vi "ixonScan.vi"(8 "stageReturnPosition":string, 9 "goBackAfterScan":bool=TRUE, 10 "scanStep":dbl, 11 "scanLength":dbl=25.0) -> (2 "Right Graph":i32[][](graph) caption="Object Image", 3 "imageCube":i32[][][](array[numeric]))   [LabVIEW 2016]
uses:
  <userlib>/atmcd64d.llb/Error Code Enum typedef.ctl
  <vilib>/Instr/_visa.llb/VISA Configure Serial Port (Instr).vi
  variables/imageSettings.vi
  variables/configDB.vi
panel:
  in  "Scan Abort":bool
  out "relative seconds 2":dbl format="%_19f"
  out "relative seconds":dbl format="%_19f"
  out "Constructing data":u8(slide) scale=0.0..256.0
  out "x-y":dbl
  out "Total \nScan Frame":dbl
  out "Current \nScan Frame":dbl
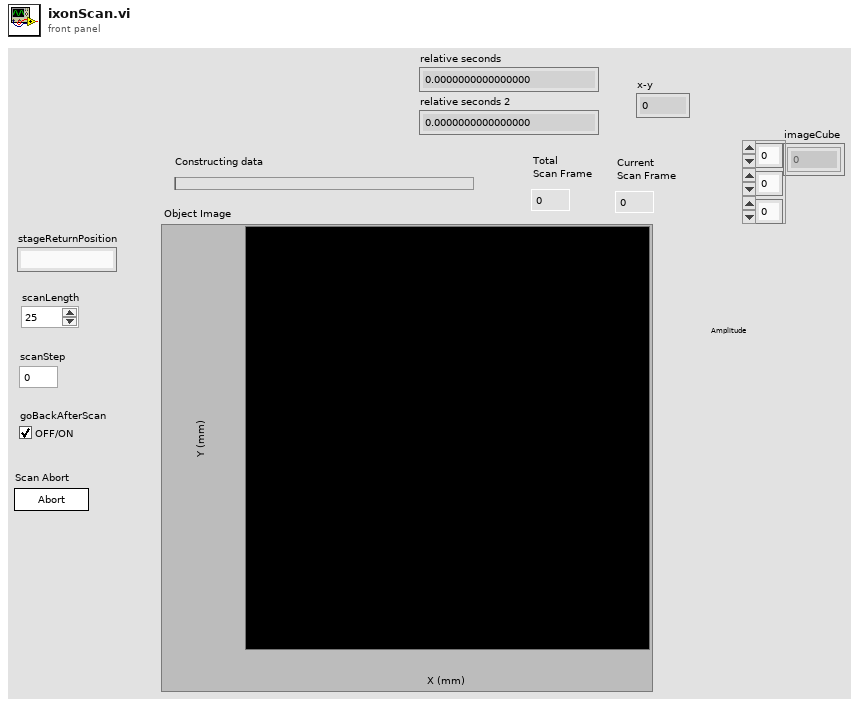
[diagram p1: front panel]
types:
  T1 = typedef "Error Code Enum typedef.ctl" = enum32{"N/A (0)", "DRV_ERROR_CODES", "DRV_SUCCESS", "DRV_VXDNOTINSTALLED", "DRV_ERROR_SCAN", "DRV_ERROR_CHECK_SUM", "DRV_ERROR_FILELOAD", "DRV_UNKNOWN_FUNC", "DRV_ERROR_VXD_INIT", "DRV_ERROR_ADDRESS", "DRV_ERROR_PAGELOCK", "DRV_ERROR_PAGEUNLOCK", "DRV_ERROR_BOARDTEST", "DRV_ERROR_ACK", "DRV_ERROR_UP_FIFO", "DRV_ERROR_PATTERN", "N/A (16)", "DRV_ACQUISITION_ERRORS", "DRV_ACQ_BUFFER", "DRV_ACQ_DOWNFIFO_FULL", "DRV_PROC_UNKONWN_INSTRUCTION", "DRV_ILLEGAL_OP_CODE", "DRV_KINETIC_TIME_NOT_MET", "DRV_ACCUM_TIME_NOT_MET", "DRV_NO_NEW_DATA", "N/A (25)", "DRV_SPOOLERROR", "N/A (27)", "N/A (28)", "N/A (29)", "N/A (30)", "N/A (31)", "N/A (32)", "DRV_TEMPERATURE_CODES", "DRV_TEMPERATURE_OFF", "DRV_TEMPERATURE_NOT_STABILIZED", "DRV_TEMPERATURE_STABILIZED", "DRV_TEMPERATURE_NOT_REACHED", "DRV_TEMPERATURE_OUT_RANGE", "DRV_TEMPERATURE_NOT_SUPPORTED", "DRV_TEMPERATURE_DRIFT", "N/A (41)", "N/A (42)", "N/A (43)", "N/A (44)", "N/A (45)", "N/A (46)", "N/A (47)", "N/A (48)", "DRV_GENERAL_ERRORS", "DRV_INVALID_AUX", "DRV_COF_NOTLOADED", "DRV_FPGAPROG", "DRV_FLEXERROR", "DRV_GPIBERROR", "N/A (55)", "N/A (56)", "N/A (57)", "N/A (58)", "N/A (59)", "N/A (60)", "N/A (61)", "N/A (62)", "N/A (63)", "DRV_DATATYPE", "DRV_DRIVER_ERRORS", "DRV_P1INVALID", "DRV_P2INVALID", "DRV_P3INVALID", "DRV_P4INVALID", "DRV_INIERROR", "DRV_COFERROR", "DRV_ACQUIRING", "DRV_IDLE", "DRV_TEMPCYCLE", "DRV_NOT_INITIALIZED", "DRV_P5INVALID", "DRV_P6INVALID", "DRV_INVALID_MODE", "DRV_INVALID_FILTER", "DRV_I2CERRORS", "DRV_I2CDEVNOTFOUND", "DRV_I2CTIMEOUT", "DRV_P7INVALID", "N/A (84)", "N/A (85)", "N/A (86)", "N/A (87)", "N/A (88)", "N/A (89)", "DRV_IOCERROR", "DRV_VRMVERSIONERROR"}
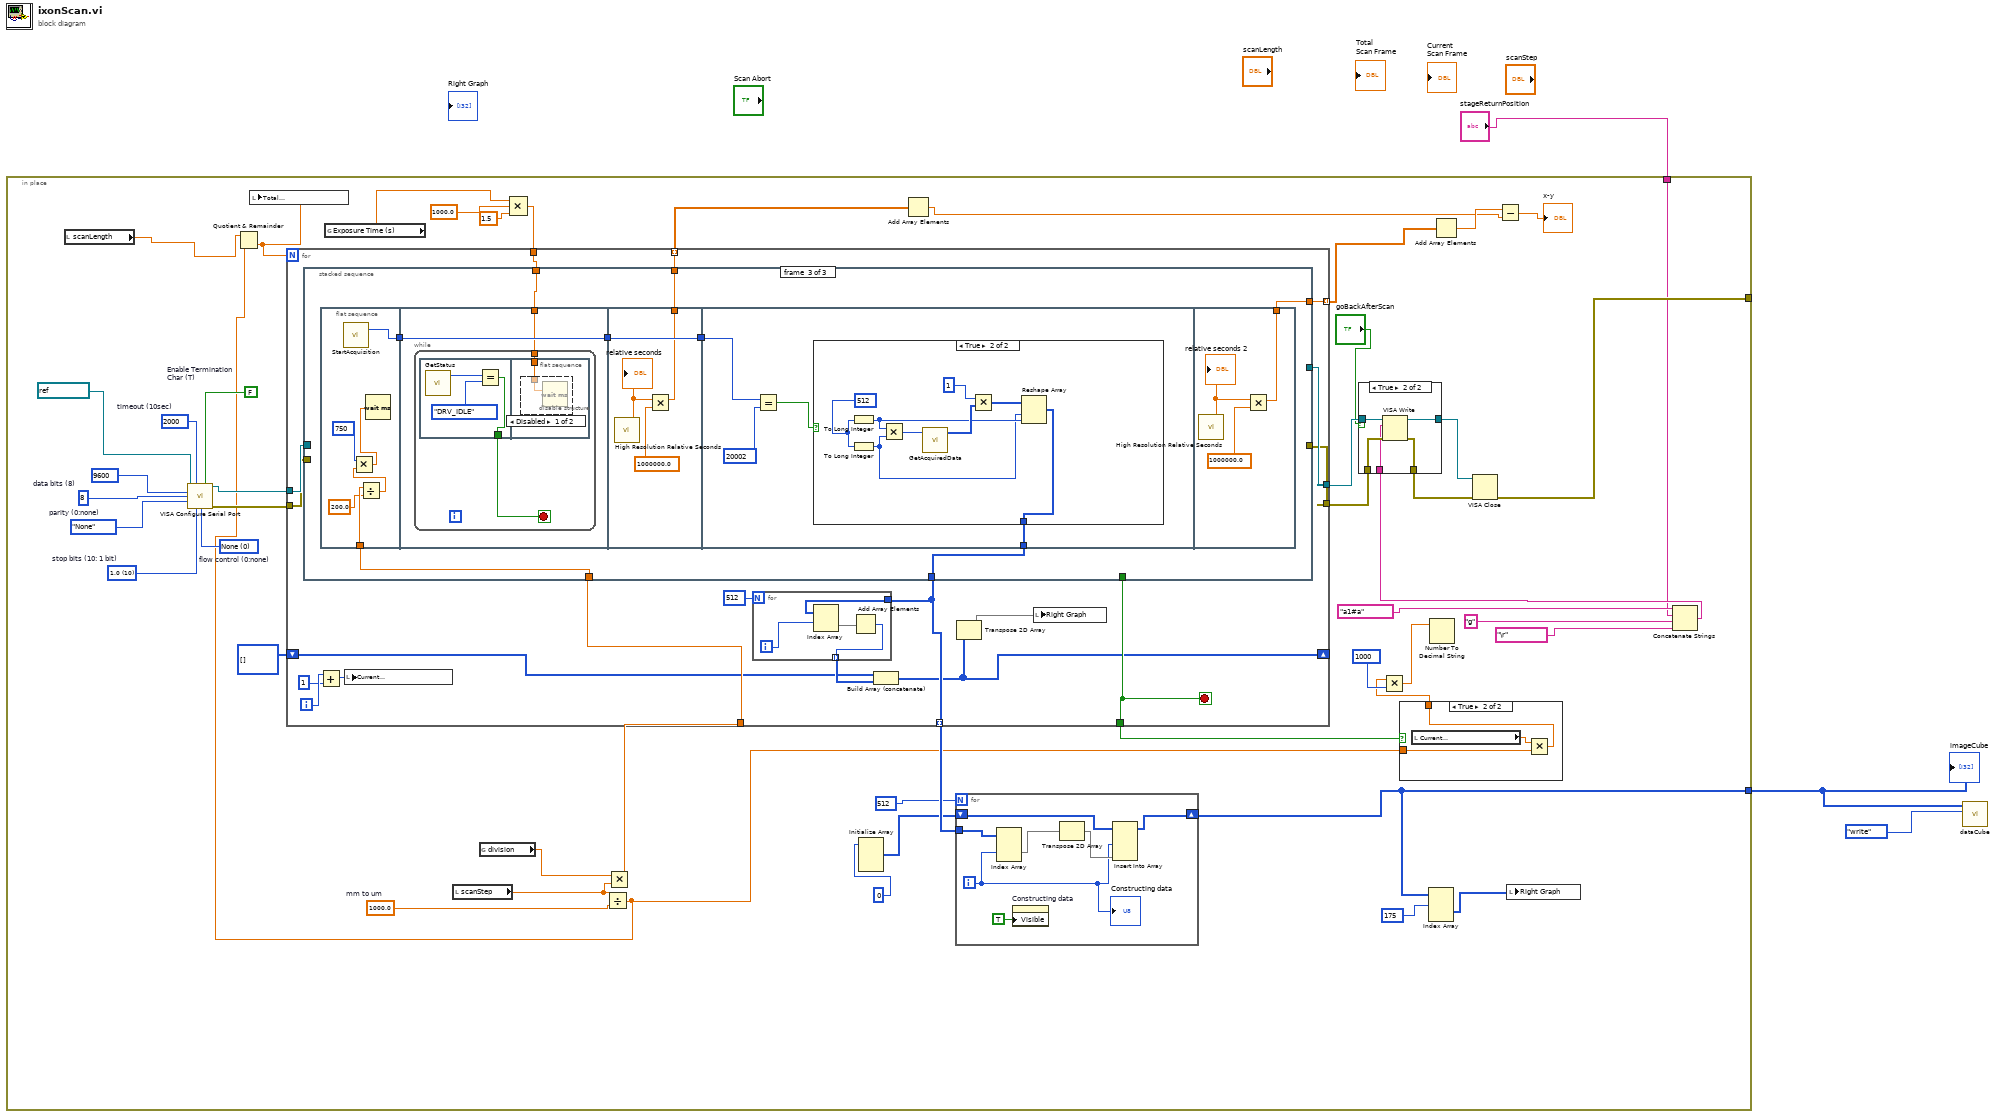
[diagram p0: block diagram]
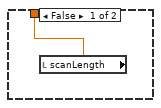
[diagram p3: hidden frame]
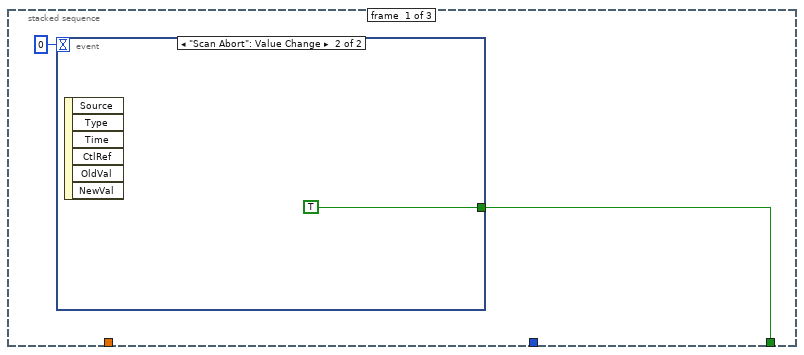
[diagram p4: hidden frame]
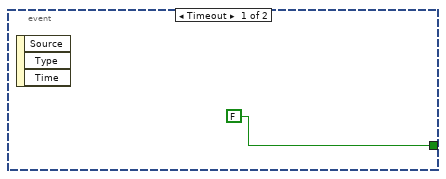
[diagram p5: hidden frame]
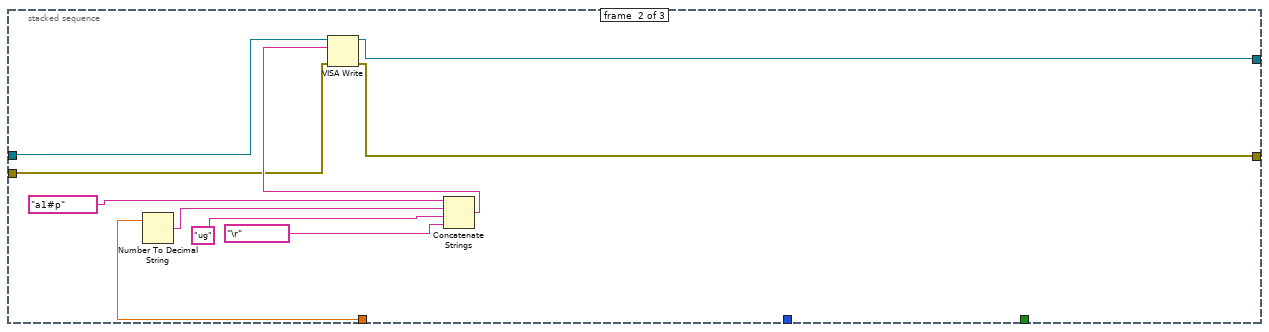
[diagram p6: hidden frame]
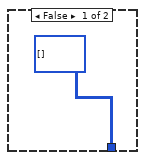
[diagram p8: hidden frame]
diagram:
  n1 = in-place {
    in-place-border: [w30] -> _
    in-place-border: [w24] -> w1
    in-place-border: "stageReturnPosition" -> [w17]
    w21 = 1000.0  # mm to um
    w46 = u16 0 items=["None", "XON/XOFF", "RTS/CTS", "XON/XOFF & RTS/CTS", "DTR/DSR", "XON/XOFF & DTR/DSR"]  # flow control (0:none)
    w47 = u16 10 items=["1.0"=10, "1.5"=15, "2.0"=20]  # stop bits (10: 1 bit)
    w48 = FALSE  # Enable Termination Char (T)
    w49 = u32 2000  # timeout (10sec)
    w50 = enum16{"None", "Odd", "Even", "Mark", "Space"}."None"  # parity (0:none)
    w51 = u16 8  # data bits (8)
    n2 = local read "scanLength"() -> (w12:dbl)
    n3 = call-poly "VISA Configure Serial Port"("VISA resource name"=refnum<visa-resource-name> "COM4", "timeout (10sec)"=w49, "Enable Termination\nChar (T)"=w48, "baud rate (9600)"=u32 9600, "data bits (8)"=w51, "parity (0:none)"=w50, "stop bits (10: 1 bit)"=w47, "flow control (0:none)"=w46) -> ("VISA resource name out"=w44:refnum<visa-resource-name>, "error out"=w43:errorcluster)  [unwired: 6 in]
    n4 = global read "imageSettings.vi" "Exposure Time (s)"() -> (w5:sgl)
    n5 = local read "scanStep"() -> (w20:dbl)
    n6 = global read "configDB.vi" "division"() -> (w4:dbl)
    n7 = Compound Arithmetic op=MULTIPLY(w5, sgl 1000.0 ("y"), sgl 1.5 ("value")) -> (w27:sgl)
    n8 = Divide(x=w20, y=w21) -> (x/y=w11:dbl)
    n9 = Quotient & Remainder(x=w12, y=w11) -> (floor(x/y)=w13:dbl)  [unwired: 1 out]
    n10 = local write "Total \nScan Frame"(w13) -> ()
    n11 = Multiply(x=w4, y=w20) -> (x*y=w14:dbl)
    n12 = for {
      N: w13 -> [_]
      tunnel: w44 -> [w88]
      tunnel: w43 -> [w87]
      tunnel: [w85] -> w42
      tunnel: [w84] -> w41
      tunnel: [w78] -> w35 mode=indexing
      tunnel: w14 -> [w86]
      tunnel: w27 -> [w83]
      tunnel: [w81] -> w26
      shift-right: [w74] -> _
      shift-left: i32[][] [] -> [w75]
      tunnel: [w72] -> w6 mode=indexing
      tunnel: [w71] -> w7 mode=indexing
      i -> [w82]
      stop <- w81 stop-if-true
      n13 = stacked-sequence {
        tunnel: w88 -> [_ w105 _]
        tunnel: w87 -> [_ w104 _]
        tunnel: [_ w98 _] -> w85
        tunnel: [_ _ w113] -> w78
        tunnel: w86 -> [_ w99 w111]
        tunnel: [_ w97 _] -> w84
        tunnel: w83 -> [_ _ w112]
        tunnel: [w93 _ _] -> w81
        tunnel: [_ _ w108] -> w72
        tunnel: [_ _ w107] -> w71
        frame #0 {
          n14 = event shown="[1] \"Scan Abort\": Value Change" {
            selector: _ -> [_ _]
            dyn-events: _ -> [_ _]
            timeout: 0 -> [_ _]
            tunnel: [FALSE TRUE] -> w93
            event Timeout {
              n15 = event-data() -> ()  [unwired: 1 in, 3 out]
            }
            event "Scan Abort": Value Change {
              n16 = event-data() -> ()  [unwired: 1 in, 6 out]
            }
          }
        }
        frame #1 {
          n17 = Number To Decimal String(number=w99) -> (decimal integer string=w100:string)  [unwired: 1 in]
          n18 = Concatenate Strings("a1#p" ("string"), w100, "ug" ("string"), "\r" ("write buffer")) -> (w106:string)
          n19 = VISA Write(VISA resource name=w105, write buffer=w106, error in (no error)=w104) -> (VISA resource name out=w98:refnum<visa-resource-name>, error out=w97:errorcluster)  [unwired: 1 out]
        }
        frame #2 {
          n20 = flat-sequence {
            tunnel: [w120] -> w114
            tunnel: w111 -> [w119]
            tunnel: w114 -> [w122]
            tunnel: [w122] -> w110
            tunnel: w112 -> [w121]
            tunnel: w110 -> [w133]
            tunnel: [w133] -> w109
            tunnel: [w131] -> w107
            tunnel: w109 -> [w137]
            tunnel: [w134] -> w113
            tunnel: [w148] -> w108
            frame #0 {
              n21 = call <userlib>:"StartAcquisition.vi"() -> ("DLL error code"=w120:u32)  [unwired: 2 in, 1 out]
              n22 = Divide(x=w119, y=200.0) -> (x/y=w116:dbl)
              n23 = Multiply(x=u32 750 ("milliseconds to wait"), y=w116) -> (x*y=w115:dbl)
              n24 = Wait (ms)(milliseconds to wait=w115) -> ()  [unwired: 1 out]
            }
            frame #1 {
              n25 = while {
                tunnel: w121 -> [w123]
                stop <- w124 stop-if-true
                n26 = flat-sequence {
                  tunnel: [w125] -> w124
                  tunnel: w123 -> [w128]
                  frame #0 {
                    n27 = call <userlib>:"GetStatus.vi"() -> ("status"=w126:T1)  [unwired: 3 in, 2 out]
                    n28 = Equal?(x=w126, y=Error_Code_Enum_typedef."DRV_IDLE" ("status")) -> (x = y?=w125:bool)
                  }
                  frame #1 {
                    n29 = disable-structure shown="Disabled" {
                      disable-tunnel: w128 -> [w129 _]
                      frame Disabled {
                        n30 = Wait (ms)(milliseconds to wait=w129) -> ()  [unwired: 1 out]
                      }
                      frame Enabled {
                      }
                    }
                  }
                }
              }
            }
            frame #2 {
              n31 = call <vilib>:"High Resolution Relative Seconds.vi"() -> ("relative seconds"=w132:dbl)
              "relative seconds" <- w132
              n32 = Multiply(x=w132, y=1000000.0) -> (x*y=w131:dbl)
            }
            frame #3 {
              n33 = Equal?(x=w137, y=u32 20002) -> (x = y?=w135:bool)
              n34 = case shown="True" w135 {
                tunnel: [i32[][] [] w139] -> w134
                frame False {
                }
                frame True {
                  w140 = 512
                  n35 = To Long Integer(number=w140) -> (32bit integer=w142:i32)
                  n36 = To Long Integer(number=w140) -> (32bit integer=w141:i32)
                  n37 = Multiply(x=w142, y=w141) -> (x*y=w146:i32)
                  n38 = call <userlib>:"GetAcquiredData.vi"("size"=w146) -> ("array"=w144:i32[])  [unwired: 2 in, 2 out]
                  n39 = Multiply(x=1, y=w144) -> (x*y=w143:i32[])
                  n40 = Reshape Array(w143, w141, w142) -> (w139:i32[][])
                }
              }
            }
            frame #4 {
              n41 = call <vilib>:"High Resolution Relative Seconds.vi"() -> ("relative seconds"=w149:dbl)
              "relative seconds 2" <- w149
              n42 = Multiply(x=w149, y=1000000.0) -> (x*y=w148:dbl)
            }
          }
        }
      }
      n43 = Add(x=w82, y=1) -> (x+y=w80:i32)
      n44 = local write "Current \nScan Frame"(w80) -> ()
      n45 = for {
        N: 512 -> [_]
        tunnel: w78 -> [w92]
        tunnel: [w89] -> w76 mode=indexing
        i -> [w91]
        n46 = Index Array(array=w92, index (row)=w91) -> (element=w90:i32[])  [unwired: 1 in]
        n47 = Add Array Elements(numeric array=w90) -> (sum=w89:i32)
      }
      n48 = Build Array (concatenate)(w75, w76) -> (w74:i32[][])
      n49 = Transpose 2D Array(2D array=w74) -> (transposed array=w73:i32[][])
      n50 = local write "Right Graph"(w73) -> ()
    }
    n51 = Initialize Array(0 ("element")) -> (w32:i32[][][])  [unwired: 3 in]
    n52 = Add Array Elements(numeric array=w7) -> (sum=w9:dbl)
    n53 = for {
      N: 512 -> [_]
      tunnel: w35 -> [w70]
      shift-right: [w67] -> w24
      shift-left: w32 -> [w66]
      i -> [w64]
      n54 = Index Array(array=w70, index (dim 1)=w64) -> (element=w69:i32[][])  [unwired: 2 in]
      n55 = property on="Constructing data" class="Slide (strict)"("Visible"=TRUE) -> ()  [unwired: 2 in, 2 out]
      n56 = Transpose 2D Array(2D array=w69) -> (transposed array=w68:i32[][])
      n57 = Insert Into Array(array=w66, index (dim 1)=w64, new element=w68) -> (w67:i32[][][])  [unwired: 2 in]
      "Constructing data" <- w64
    }
    n58 = case shown="True" w26 {
      tunnel: [w60 w62] -> w25
      tunnel: w11 -> [_ w61]
      frame False {
        n59 = local read "scanLength"() -> (w60:dbl)
      }
      frame True {
        n60 = local read "Current \nScan Frame"() -> (w63:dbl)
        n61 = Multiply(x=w63, y=w61) -> (x*y=w62:dbl)
      }
    }
    n62 = Multiply(x=w25, y=1000) -> (x*y=w36:dbl)
    n63 = Index Array(array=w24, index (dim 0)=175 ("index (page)")) -> (element=w22:i32[][])  [unwired: 2 in]
    n64 = Number To Decimal String(number=w36) -> ()  [unwired: 1 in, 1 out]
    n65 = Add Array Elements(numeric array=w6) -> (sum=w10:dbl)
    n66 = Subtract(x=w10, y=w9) -> (x-y=→"x-y":dbl)
    n67 = local write "Right Graph"(w22) -> ()
    n68 = Concatenate Strings("a1#a" ("string"), w17, "g" ("string"), "\r" ("write buffer")) -> (w37:string)
    n69 = case shown="True" "goBackAfterScan" {
      tunnel: w42 -> [w54 w59]
      tunnel: w41 -> [w53 w58]
      tunnel: [w53 w57] -> w40
      tunnel: [w54 w56] -> w39
      tunnel: w37 -> [_ w55]
      frame False {
      }
      frame True {
        n70 = VISA Write(VISA resource name=w59, write buffer=w55, error in (no error)=w58) -> (VISA resource name out=w56:refnum<visa-resource-name>, error out=w57:errorcluster)  [unwired: 1 out]
      }
    }
    n71 = VISA Close(VISA resource name=w39, error in (no error)=w40) -> (error out=w30:errorcluster)
  }
  "imageCube" <- w1
  n72 = call "dataCube.vi"("Enum"=enum16{"clear", "read", "write"}."write", "imageCube"=w1) -> ()  [unwired: 9 in, 1 out]
